vi "Test_WriteValue_CheckTerminal_TerminalUpdated.vi"(8 "error in (no error)":errorcluster, 11 "TestCase in":refnum<class "TestTerminalSignalingValueBinding.lvclass">) -> (0 "error out":errorcluster, 3 "TestCase out":refnum<class "TestTerminalSignalingValueBinding.lvclass">)   [LabVIEW 2017, in "TestTerminalSignalingValueBinding.lvclass"]
uses:
  TestTerminalSignalingValueBinding.lvclass
  Source/Concrete/TerminalSignalingValueBinding/TerminalSignalingValueBinding.lvclass
  C:/Git/composed-transport/Source/ITransport/ITransport.lvclass
  Source/ITransport/ITransport.lvclass
panel:
  in  "Numeric":i32
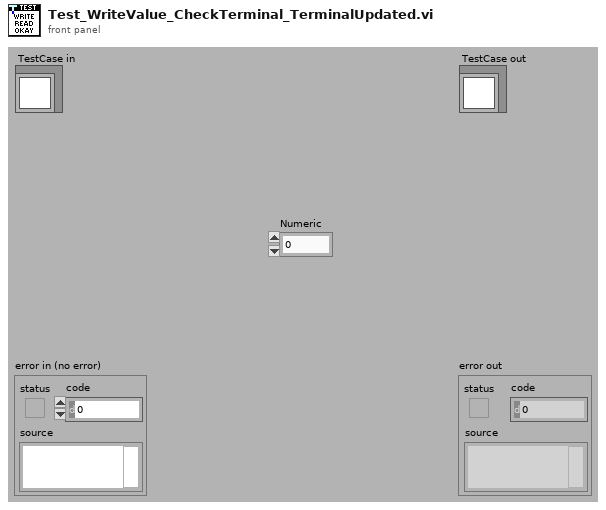
[diagram p1: front panel]
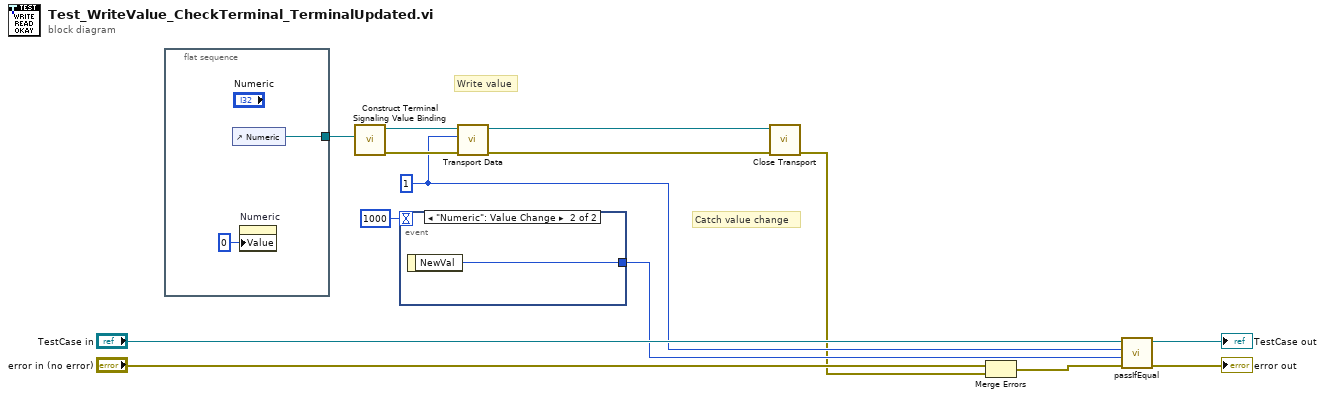
[diagram p0: block diagram]
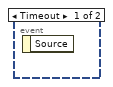
[diagram p2: hidden frame]
diagram:
  w3 = 1
  # "Catch value change"
  # "Write value"
  n1 = flat-sequence {
    tunnel: [w16] -> w6
    frame #0 {
      n2 = control-ref of="Numeric"() -> (w16:refnum<vi>)
      n3 = property on="Numeric" class="DigNum (strict)"("Value"=0 ("Numeric")) -> ()  [unwired: 2 in, 2 out]
    }
  }
  n4 = call "Construct Terminal Signaling Value Binding.vi"("Ctl Refnum"=w6) -> ("error out"=w14:errorcluster, "TerminalSignalingValueBinding"=w9:refnum<class "TerminalSignalingValueBinding.lvclass">)  [unwired: 9 in]
  n5 = event shown="[1] \"Numeric\": Value Change" {
    selector: _ -> [_ _]
    dyn-events: _ -> [_ _]
    timeout: 1000 -> [_ _]
    tunnel: [_ w17] -> w2
    event Timeout {
      n6 = event-data() -> ()  [unwired: 1 in, 1 out]
    }
    event "Numeric": Value Change {
      n7 = event-data() -> ("NewVal"=w17:i32)  [unwired: 1 in]
    }
  }
  n8 = call "Transport Data.vi"("error in (no error)"=w14, "Value"=w3, "ITransport in"=w9) -> ("error out"=w5:errorcluster, "ITransport out"=w7:refnum<class "TerminalSignalingValueBinding.lvclass">)  [unwired: 7 in]
  n9 = call-dynamic "Close Transport.vi"("error in (no error)"=w5, "ITransport in"=w7) -> ("error out"=w1:errorcluster)  [unwired: 9 in]
  n10 = Merge Errors("error in (no error)", w1) -> (w8:errorcluster)
  n11 = call-dynamic "passIfEqual.vi"("error in (no error)"=w8, "y"=w2, "x"=w3, "TestCase in"="TestCase in") -> ("error out"=→"error out":errorcluster, "TestCase out"=→"TestCase out":refnum<class "TestTerminalSignalingValueBinding.lvclass">)  [unwired: 6 in]
